vi "Rotating a Picture.vi"() -> ()   [LabVIEW 2016]
doc: "Demonstrates how to rotate an image displayed in a 2D Picture. This feature is important when you want to animate the state of an object, like the attitude of an airplane."
uses:
  <vilib>/picture/picture.llb/Draw True-Color Pixmap.vi
panel:
  in  "Stop":bool
  in  "Rotation Angle (radians)":dbl(knob) scale=-3.14..3.14
  out "2D Picture":picture
  # "Overview: This VI demonstrates how to rotate an image displayed in a 2D Picture.\nInstructions: \n1. Run the VI. \n2. Change the Rotation Angle of the image and observe the change in the displayed image.\n3. Click Stop to stop the VI."
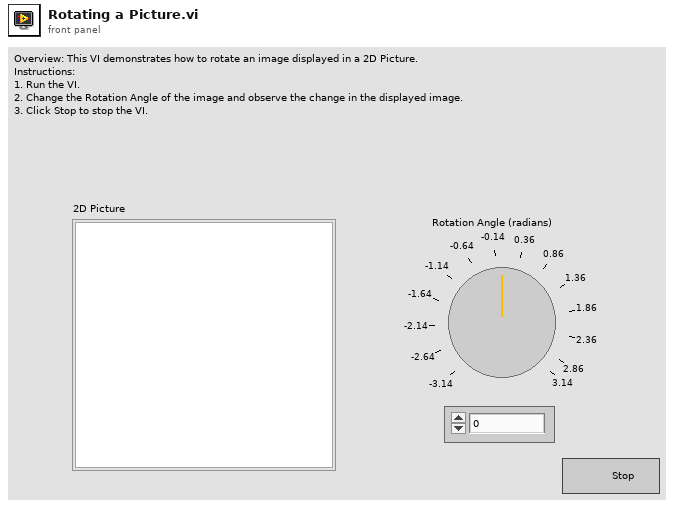
[diagram p1: front panel]
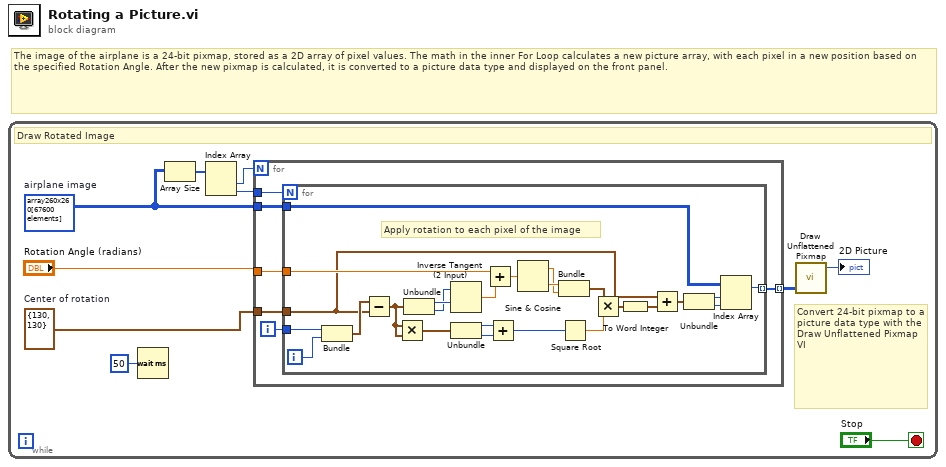
[diagram p0: block diagram]
diagram:
  # "The image of the airplane is a 24-bit pixmap, stored as a 2D array of pixel values. The math in the inner For Loop calculates a new picture array, with each pixel in a new position based on the specified Rotation Angle. After the new pixmap is calculated, it is converted to a picture data type and displayed on the front panel."
  n1 = while {
    stop <- "Stop" stop-if-true
    w6 = u32[][] array260x260[67600 elements]  # airplane image
    w4 = cluster{"x":i16, "y":i16} {"x"=130, "y"=130}  # Center of rotation
    # "Convert 24-bit pixmap to a picture data type with the Draw Unflattened Pixmap VI"
    # "Draw Rotated Image"
    n2 = Wait (ms)(milliseconds to wait=u32 50) -> ()  [unwired: 1 out]
    n3 = Array Size(array=w6) -> (size(s)=w10:i32[])
    n4 = Index Array(array=w10) -> (element #1=w8:i32, element #2=w9:i32)  [unwired: 2 in]
    n5 = for {
      N: w8 -> [_]
      tunnel: w9 -> [w15]
      tunnel: w4 -> [w14]
      tunnel: "Rotation Angle (radians)" -> [w13]
      tunnel: w6 -> [w12]
      tunnel: [w11] -> w7 mode=indexing
      i -> [w16]
      n6 = for {
        N: w15 -> [_]
        tunnel: w16 -> [w41]
        tunnel: w14 -> [w19]
        tunnel: w13 -> [w30]
        tunnel: w12 -> [w20]
        tunnel: [w18] -> w11 mode=indexing
        i -> [w40]
        # "Apply rotation to each pixel of the image"
        n7 = Bundle(w41, w40) -> (w39:cluster{i32, i32})  [unwired: 1 in]
        n8 = Subtract(x=w39, y=w19) -> (x-y=w34:cluster{i32, i32})
        n9 = Multiply(x=w34, y=w34) -> (x*y=w38:cluster{i32, i32})
        n10 = Unbundle(w34) -> (w33:i32, w32:i32)
        n11 = Inverse Tangent (2 Input)(1:w33, 2:w32) -> (0:w31:dbl)
        n12 = Unbundle(w38) -> (w37:i32, w36:i32)
        n13 = Add(x=w30, y=w31) -> (x+y=w29:dbl)
        n14 = Add(x=w37, y=w36) -> (x+y=w35:i32)
        n15 = Sine & Cosine(0:w29) -> (1:w27:dbl, 2:w28:dbl)
        n16 = Bundle(w28, w27) -> (w26:cluster{dbl, dbl})  [unwired: 1 in]
        n17 = Square Root(x=w35) -> (sqrt(x)=w25:dbl)
        n18 = Multiply(x=w26, y=w25) -> (x*y=w24:cluster{dbl, dbl})
        n19 = To Word Integer(number=w24) -> (16bit integer=w23:cluster{i16, i16})
        n20 = Add(x=w19, y=w23) -> (x+y=w17:cluster{i16, i16})
        n21 = Unbundle(w17) -> (w22:i16, w21:i16)
        n22 = Index Array(array=w20, index (row)=w22, index (col)=w21) -> (element=w18:u32)
      }
    }
    n23 = call-poly <vilib>:"Draw Unflattened Pixmap.vi"("data (RGB format)"=w7) -> ("new picture"=→"2D Picture":picture)  [unwired: 8 in]
  }
